vi "Get Property Name.vi"(8 "error in":errorcluster, 11 "Property Node in":refnum<k20>) -> (0 "error out":errorcluster, 2 "Property Value":string, 3 "Property Node out":refnum<k20>)   [LabVIEW 2024, in "Config File Parser.lvlib" / "Property.lvclass"]
uses:
  Property.lvclass
  <vilib>/xml/Close Reference(Node).vi
  <resource>/objmgr/DOMUserDefRef.rc
  <vilib>/xml/NI_XML.lvlib
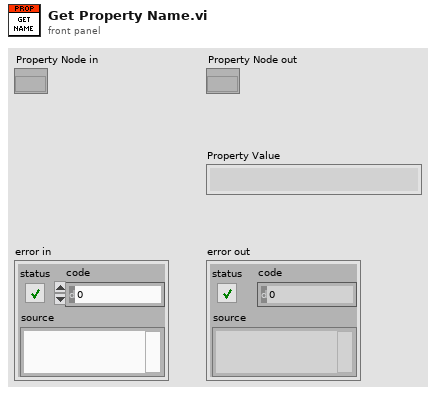
[diagram p1: front panel]
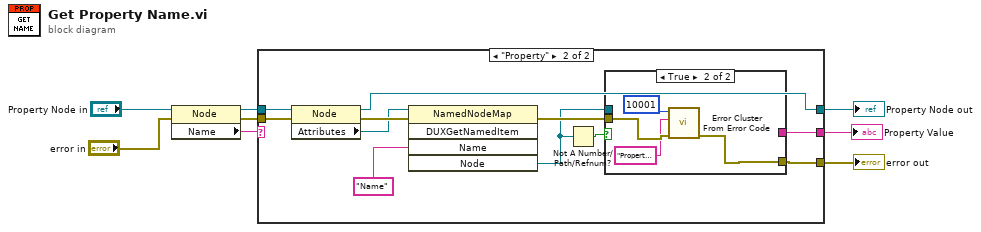
[diagram p0: block diagram]
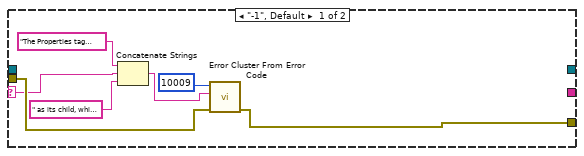
[diagram p2: hidden frame]
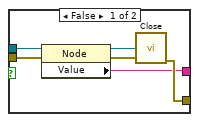
[diagram p3: hidden frame]
diagram:
  n1 = property class="Node"(reference="Property Node in", error in="error in") -> (reference out=w3:refnum<k20>, error out=w6:errorcluster, "Name"=w2:string)
  n2 = case shown="\"Property\"" w2 {
    selector: w2 -> [w10 _]
    tunnel: w3 -> [_ w22]
    tunnel: [_ w20] -> w4
    tunnel: w6 -> [w15 w26]
    tunnel: [w14 w23] -> w8
    tunnel: [_ w16] -> w1
    frame "-1", Default {
      n3 = Concatenate Strings("The Properties tag should only contain Property as its child. Here Properties tag contains " ("Additional Message"), w10, " as its child, which is not acceptable." ("string")) -> (w12:string)
      n4 = call <vilib>:"Error Cluster From Error Code.vi"("error in (no error)"=w15, "error message (\"\")"=w12, "error code (0)"=10009 ("Code")) -> ("error out"=w14:errorcluster)  [unwired: 6 in]
    }
    frame "Property" {
      n5 = property class="Node"(reference=w22, error in=w26) -> (reference out=w16:refnum<k20>, error out=w25:errorcluster, "Attributes"=w21:refnum<k20>)
      n6 = invoke class="NamedNodeMap" method="DUXGetNamedItem"(reference=w21, error in=w25, "Name"="Name") -> (error out=w24:errorcluster, "Node"=w17:refnum<k20>)  [unwired: 2 in, 3 out]
      n7 = Not A Number/Path/Refnum?(number/path/refnum=w17) -> (NaN/Path/Refnum?=w18:bool)
      n8 = case shown="True" w18 {
        tunnel: w17 -> [w29 _]
        tunnel: [w28 _] -> w20
        tunnel: w24 -> [w32 w35]
        tunnel: [w30 w36] -> w23
        frame False {
          n9 = property class="Node"(reference=w29, error in=w32) -> (reference out=w27:refnum<k20>, error out=w31:errorcluster, "Value"=w28:string)
          n10 = call-poly <vilib>:"Close.vi"("error in (no error)"=w31, "node"=w27) -> ("error out"=w30:errorcluster)  [unwired: 7 in]
        }
        frame True {
          n11 = call <vilib>:"Error Cluster From Error Code.vi"("error in (no error)"=w35, "error message (\"\")"="Property should have a name attribute", "error code (0)"=10001) -> ("error out"=w36:errorcluster)  [unwired: 6 in]
        }
      }
    }
  }
  "Property Value" <- w4
  "error out" <- w8
  "Property Node out" <- w1
